vi "Render.vi"(8 "error in (no error)":errorcluster, 11 "Line in":refnum<class "Line.lvclass">) -> (0 "error out":errorcluster, 2 "Picture Bckgnd":picture, 3 "Line out":refnum<class "Line.lvclass">)   [LabVIEW 2014, in "Line.lvclass"]
uses:
  Line.lvclass
  Line.lvclass/Line.ctl
  Graphic.lvclass
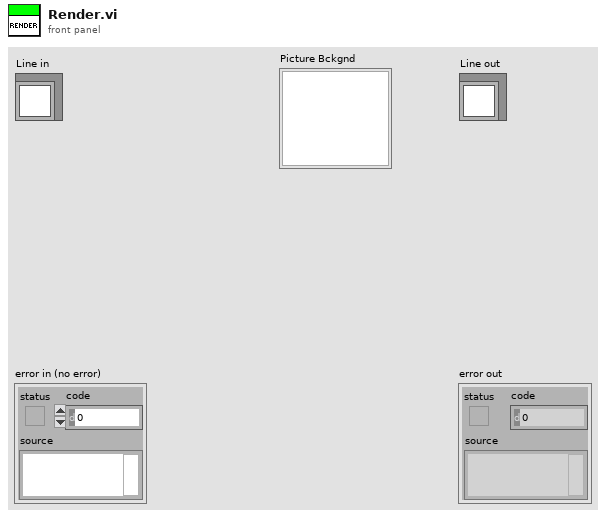
[diagram p1: front panel]
types:
  T1 = cluster{"Width":u16, "Style":enum32{"Solid", "Dash", "Dot", "DashDot", "DashDotDot"}}
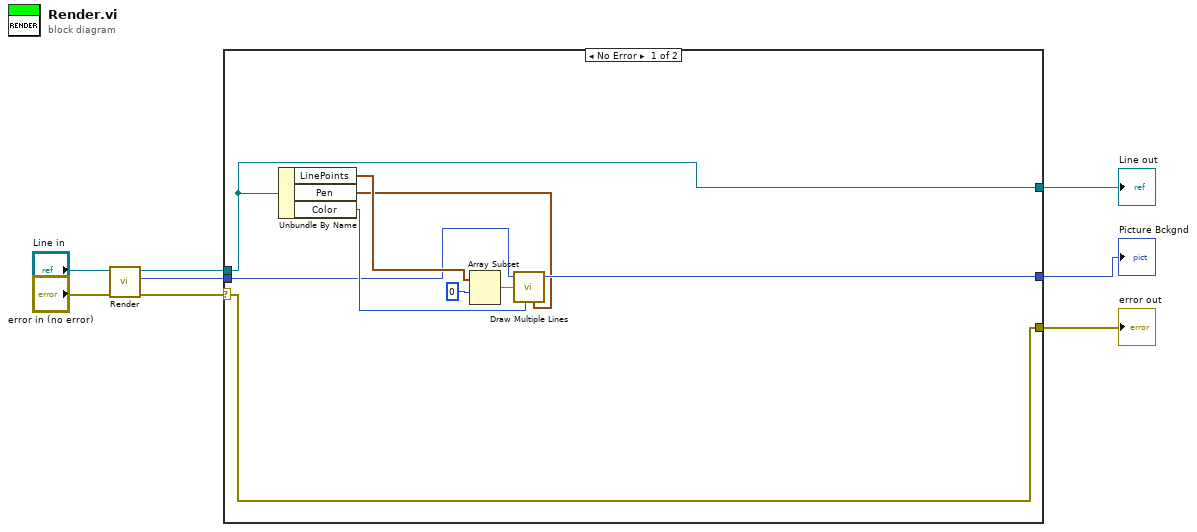
[diagram p0: block diagram]
diagram:
  n1 = call-parent "Render.vi"("error in (no error)"="error in (no error)", "Graphic in"="Line in") -> ("error out"=w6:errorcluster, "Picture Bckgnd"=w4:picture, "Graphic out"=w5:refnum<class "Line.lvclass">)  [unwired: 7 in]
  n2 = case shown="No Error" w6 {
    selector: w6 -> [w16 w18]
    tunnel: w5 -> [w10 w19]
    tunnel: w4 -> [w9 w20]
    tunnel: [w10 w19] -> w3
    tunnel: [w17 w20] -> w2
    tunnel: [w16 w18] -> w1
    frame No Error {
      n3 = Unbundle By Name(w10) -> ("LinePoints"=w15:cluster{"x":i16, "y":i16}[], "Pen"=w12:T1, "Color"=w11:u32)
      n4 = Array Subset(array=w15, index=0) -> (w13:cluster{"x":i16, "y":i16}[])  [unwired: 1 in]
      n5 = call <vilib>:"Draw Multiple Lines.vi"("picture"=w9, "line endpoints"=w13, "color(black)"=w11, "pen"=w12) -> ("new picture"=w17:picture)  [unwired: 5 in]
    }
    frame Error {
    }
  }
  "error out" <- w1
  "Line out" <- w3
  "Picture Bckgnd" <- w2
